vi "Init.vi"(3 "Container State":T3, 4 "Previous State":variant, 5 "Previous Version":T2) -> (2 "Current State":T1)   [LabVIEW 2021, in "myRIO Choice Button.xctl"]
uses:
  <vilib>/myRIO/Common/Instrument Driver Framework/Utilities/xctls/myRIO Choice Button/myRIO Choice Button.xctl
  <vilib>/myRIO/Common/Instrument Driver Framework/Utilities/xctls/myRIO Choice Button/State.ctl
  <vilib>/_xctls/Container State.ctl
  <vilib>/_xctls/Version.ctl
  <vilib>/_xctls/XControlSupport.lvlib
panel:
  in  "Default Indicator State":T1={"Title"="", "Explanation"="", "Mouse Enter Glyph"=bytes[4096], "Mouse Down Glyph"=bytes[4096], "Mouse Leave Glyph"=bytes[4096], "Mouse Enter Background"=bytes[56344], "Mouse Down Background"=bytes[56344], "Mouse Leave Background"=bytes[56344], "Button Mode"=0, "Button Square Frame"=bytes[56344], "Disabled&GrayedOut"=FALSE}
  in  "Default Control State":T1={"Title"="", "Explanation"="", "Mouse Enter Glyph"=bytes[4096], "Mouse Down Glyph"=bytes[4096], "Mouse Leave Glyph"=bytes[4096], "Mouse Enter Background"=bytes[56344], "Mouse Down Background"=bytes[56344], "Mouse Leave Background"=bytes[56344], "Button Mode"=0, "Button Square Frame"=bytes[56344], "Disabled&GrayedOut"=FALSE}
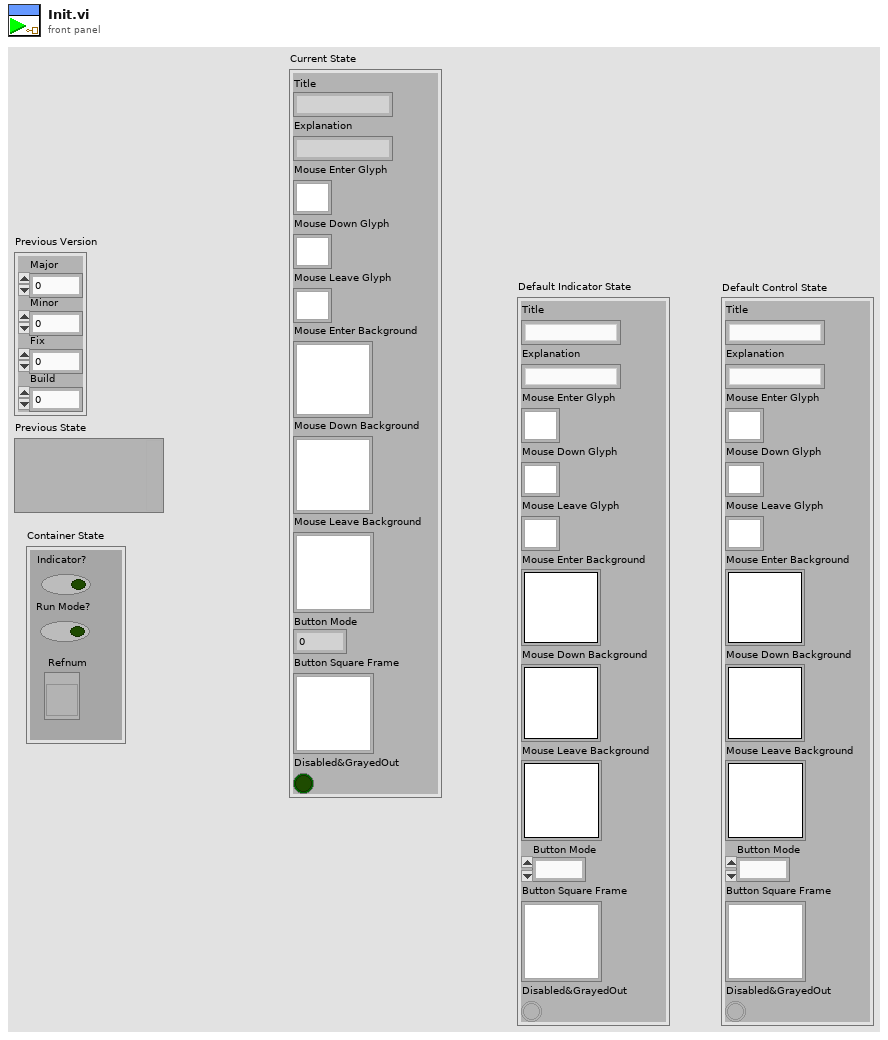
[diagram p1: front panel]
types:
  T1 = typedef "myRIO Choice Button.xctl/State.ctl" = cluster{"Title":string, "Explanation":string, "Mouse Enter Glyph":picture, "Mouse Down Glyph":picture, "Mouse Leave Glyph":picture, "Mouse Enter Background":picture, "Mouse Down Background":picture, "Mouse Leave Background":picture, "Button Mode":i32, "Button Square Frame":picture, "Disabled&GrayedOut":bool}
  T2 = typedef "XControlSupport.lvlib/Version.ctl" = cluster{"Major":u16, "Minor":u16, "Fix":u16, "Build":u16}
  T3 = typedef "XControlSupport.lvlib/Container State.ctl" = cluster{"Indicator?":bool, "Run Mode?":bool, " Refnum":refnum<vi>}
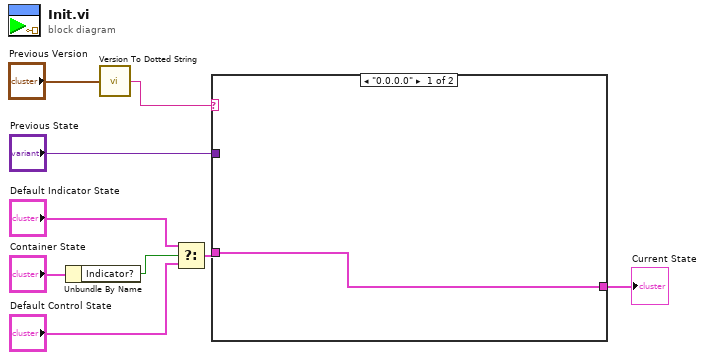
[diagram p0: block diagram]
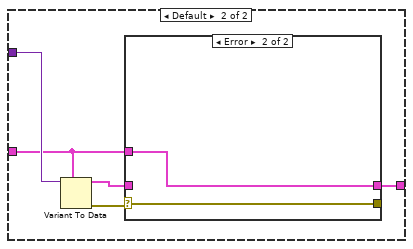
[diagram p2: hidden frame]
diagram:
  n1 = Unbundle By Name("Container State") -> ("Indicator?"=w4:bool)
  n2 = call <vilib>:"Version To Dotted String.vi"("Version"="Previous Version") -> ("String Version"=w1:string)
  n3 = Select(t="Default Indicator State", s=w4, f="Default Control State") -> (s? t:f=w3:T1)
  n4 = case shown="\"0.0.0.0\"" w1 {
    tunnel: "Previous State" -> [_ w15]
    tunnel: [w10 w11] -> w8
    tunnel: w3 -> [w10 w12]
    frame "0.0.0.0" {
    }
    frame Default {
      n5 = Variant To Data(type=w12, Variant=w15) -> (data=w13:T1, error out=w14:errorcluster)  [unwired: 1 in]
      n6 = case shown="Error" w14 {
        selector: w14 -> [w17 w18]
        tunnel: w13 -> [w16 _]
        tunnel: [w16 w19] -> w11
        tunnel: w12 -> [_ w19]
        tunnel: [w17 w18] -> _
        frame No Error {
        }
        frame Error {
        }
      }
    }
  }
  "Current State" <- w8
